vi "initialize connection object.vi"(8 "error in":errorcluster, 11 "connection":u64) -> (0 "error out":errorcluster, 3 "connection out":refnum<class "connection.lvclass">)   [LabVIEW 2016, in "connection.lvclass"]
uses:
  connection.lvclass
  connection.lvclass/connection.ctl
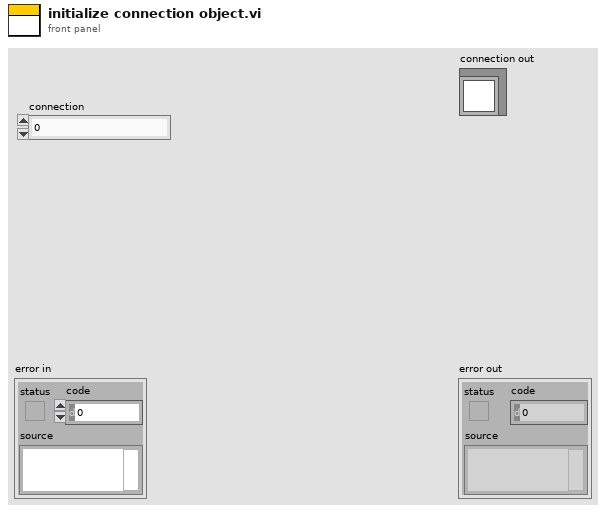
[diagram p1: front panel]
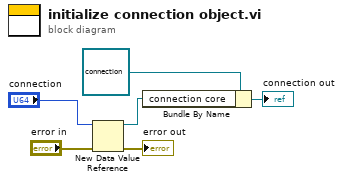
[diagram p0: block diagram]
diagram:
  n1 = New Data Value Reference(data value="connection", error in="error in") -> (data value reference=w2:refnum<data-value>, error out=→"error out":errorcluster)
  n2 = Bundle By Name(cluster=refnum<class "connection.lvclass"> refnum ("connection.lvclass"), "connection core"=w2) -> (→"connection out":refnum<class "connection.lvclass">)
